vi "Write Mouse.vi"(3 "Write Address":u8, 4 "Data In":u8, 5 "Mouse IO":T1) -> (2 "Mouse IO out":T1)   [LabVIEW 2012]
uses:
  <vilib>/rvi/eio/common/nirviEmuTemplateMethod_errors.vi
  <vilib>/eio/EIONode/EIONode.xnode
  <vilib>/eio/EIOMethodNode/EIOMethodNode.xnode
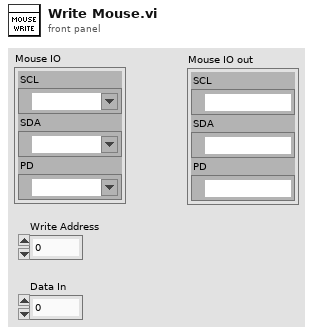
[diagram p1: front panel]
types:
  T1 = cluster{"SCL":refnum<k21>, "SDA":refnum<k21>, "PD":refnum<k21>}
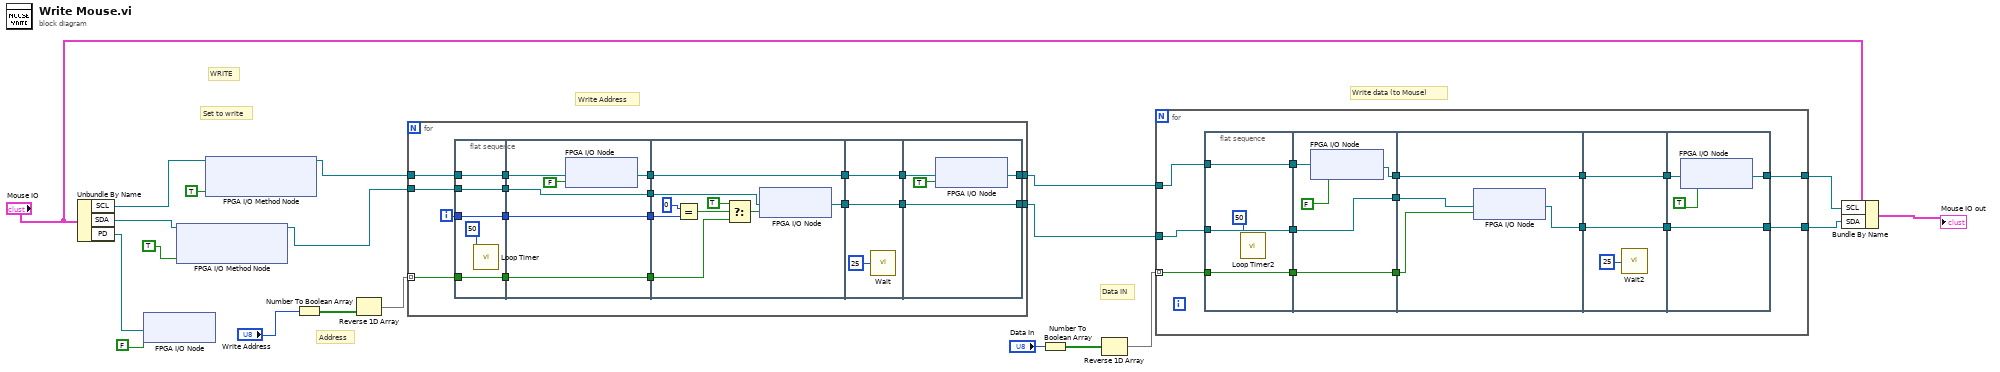
[diagram p0: block diagram]
diagram:
  # "Data IN"
  # "WRITE"
  # "Write data (to Mouse)"
  # "Write Address"
  # "Set to write"
  # "Address"
  n1 = Unbundle By Name("Mouse IO") -> ("SCL"=w6:refnum<k21>, "SDA"=w18:refnum<k21>, "PD"=w2:refnum<k21>)
  n2 = xnode "FPGA I/O Node"("I/O Item"=FALSE, "FPGA I/O In"=w2) -> ()  [unwired: 1 out]
  n3 = xnode "FPGA I/O Method Node"("FPGA I/O In"=w18, "Enable"=TRUE) -> ("FPGA I/O Out"=w8:refnum<k21>)
  n4 = xnode "FPGA I/O Method Node"("FPGA I/O In"=w6, "Enable"=TRUE) -> ("FPGA I/O Out"=w5:refnum<k21>)
  n5 = Number To Boolean Array(number="Write Address") -> (Boolean array=w19:bool[])
  n6 = Reverse 1D Array(array=w19) -> (reversed array=w7:bool[])
  n7 = for {
    tunnel: w5 -> [w38]
    tunnel: w8 -> [w35]
    tunnel: w7 -> [w31] mode=indexing
    tunnel: [w30] -> w10
    tunnel: [w29] -> w9
    i -> [w33]
    n8 = flat-sequence {
      tunnel: w31 -> [w40]
      tunnel: w33 -> [w41]
      tunnel: w35 -> [w42]
      tunnel: w38 -> [w43]
      tunnel: [w43] -> w24
      tunnel: [w42] -> w23
      tunnel: [w41] -> w22
      tunnel: [w40] -> w21
      tunnel: [w47] -> w37
      tunnel: [w46] -> w36
      tunnel: [w45] -> w34
      tunnel: [w44] -> w32
      tunnel: w24 -> [w49]
      tunnel: w23 -> [w46]
      tunnel: w22 -> [w45]
      tunnel: w21 -> [w44]
      tunnel: w37 -> [w58]
      tunnel: [w58] -> w28
      tunnel: w36 -> [w57]
      tunnel: w34 -> [w55]
      tunnel: w32 -> [w53]
      tunnel: [w50] -> w26
      tunnel: w28 -> [w61]
      tunnel: [w61] -> w27
      tunnel: w26 -> [w60]
      tunnel: [w60] -> w25
      tunnel: w27 -> [w64]
      tunnel: [w63] -> w30
      tunnel: w25 -> [w62]
      tunnel: [w62] -> w29
      frame #0 {
        n9 = call "Loop Timer"("Count(uSec)"=u16 50) -> ()  [unwired: 1 out]
      }
      frame #1 {
        n10 = xnode "FPGA I/O Node"("I/O Item"=FALSE, "FPGA I/O In"=w49) -> ("FPGA I/O Out"=w47:refnum<k21>)
      }
      frame #2 {
        n11 = Equal?(x=0 ("y"), y=w55) -> (x = y?=w56:bool)
        n12 = Select(t=TRUE, s=w56, f=w53) -> (s? t:f=w51:bool)
        n13 = xnode "FPGA I/O Node"("I/O Item"=w51, "FPGA I/O In"=w57) -> ("FPGA I/O Out"=w50:refnum<k21>)
      }
      frame #3 {
        n14 = call "Wait"("Count(uSec)"=u16 25) -> ()  [unwired: 1 out]
      }
      frame #4 {
        n15 = xnode "FPGA I/O Node"("I/O Item"=TRUE, "FPGA I/O In"=w64) -> ("FPGA I/O Out"=w63:refnum<k21>)
      }
    }
  }
  n16 = Number To Boolean Array(number="Data In") -> (Boolean array=w12:bool[])
  n17 = Reverse 1D Array(array=w12) -> (reversed array=w1:bool[])
  n18 = for {
    tunnel: w10 -> [w80]
    tunnel: w9 -> [w77]
    tunnel: w1 -> [w75] mode=indexing
    tunnel: [w74] -> w16
    tunnel: [w73] -> w15
    n19 = flat-sequence {
      tunnel: w75 -> [w82]
      tunnel: w77 -> [w83]
      tunnel: w80 -> [w84]
      tunnel: [w84] -> w72
      tunnel: [w83] -> w71
      tunnel: [w82] -> w70
      tunnel: [w87] -> w79
      tunnel: [w86] -> w78
      tunnel: [w85] -> w76
      tunnel: w72 -> [w89]
      tunnel: w71 -> [w86]
      tunnel: w70 -> [w85]
      tunnel: w79 -> [w93]
      tunnel: [w93] -> w69
      tunnel: w78 -> [w92]
      tunnel: w76 -> [w90]
      tunnel: [w91] -> w67
      tunnel: w69 -> [w96]
      tunnel: [w96] -> w68
      tunnel: w67 -> [w95]
      tunnel: [w95] -> w66
      tunnel: w68 -> [w99]
      tunnel: [w98] -> w74
      tunnel: w66 -> [w97]
      tunnel: [w97] -> w73
      frame #0 {
        n20 = call "Loop Timer2"("Count(uSec)"=u16 50) -> ()  [unwired: 1 out]
      }
      frame #1 {
        n21 = xnode "FPGA I/O Node"("I/O Item"=FALSE, "FPGA I/O In"=w89) -> ("FPGA I/O Out"=w87:refnum<k21>)
      }
      frame #2 {
        n22 = xnode "FPGA I/O Node"("I/O Item"=w90, "FPGA I/O In"=w92) -> ("FPGA I/O Out"=w91:refnum<k21>)
      }
      frame #3 {
        n23 = call "Wait2"("Count(uSec)"=u16 25) -> ()  [unwired: 1 out]
      }
      frame #4 {
        n24 = xnode "FPGA I/O Node"("I/O Item"=TRUE, "FPGA I/O In"=w99) -> ("FPGA I/O Out"=w98:refnum<k21>)
      }
    }
  }
  n25 = Bundle By Name(cluster="Mouse IO", "SCL"=w16, "SDA"=w15) -> (→"Mouse IO out":T1)
